vi "GDI Resize Image.vi"(7 "Image Data":T1, 8 "error in (no error)":errorcluster, 9 "Height":i32=400, 10 "Width":i32=800, 11 "Path":path) -> (0 "error out":errorcluster, 3 "Resized image data":T1)   [LabVIEW 2011]
doc: "Use the Windows GDI functions to resize an image."
uses:
  <vilib>/picture/picture.llb/imagedata.ctl
  System.Drawing
  <vilib>/Utility/colorconv.llb/Color to RGB.vi
  <vilib>/wsapi/NI_WebServices.lvlib
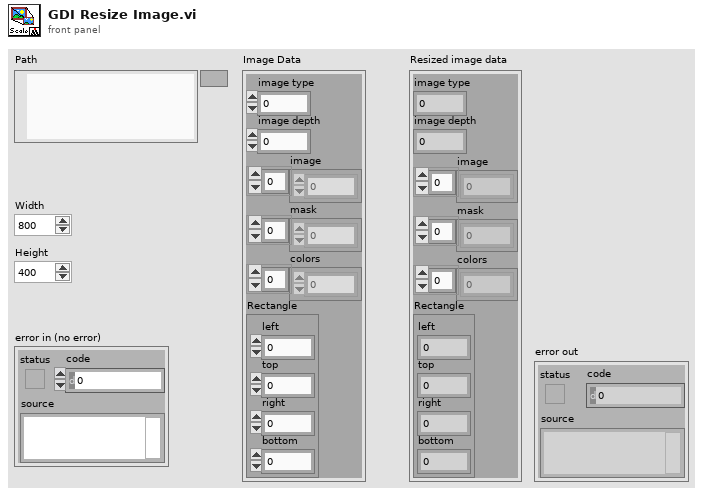
[diagram p1: front panel]
types:
  T1 = typedef "imagedata.ctl" = cluster{"image type":i32, "image depth":i32, "image":u8[], "mask":u8[], "colors":u32[], "Rectangle":cluster{"left":i16, "top":i16, "right":i16, "bottom":i16}}
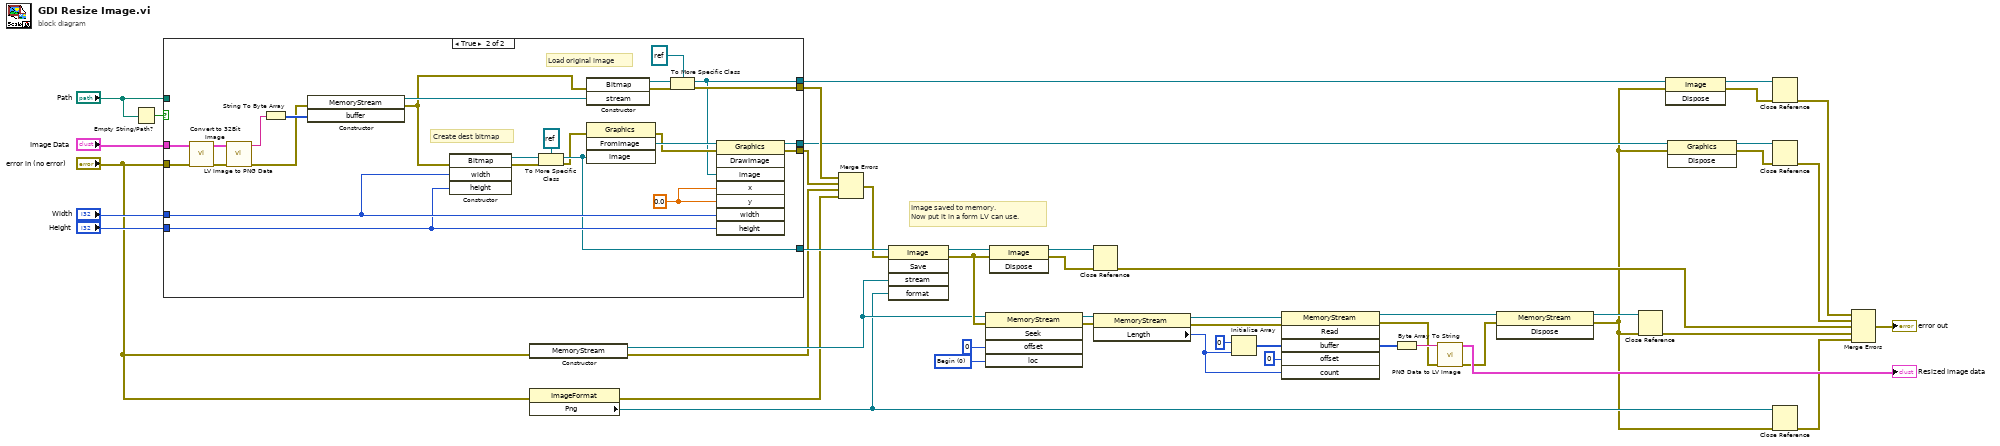
[diagram p0: block diagram]
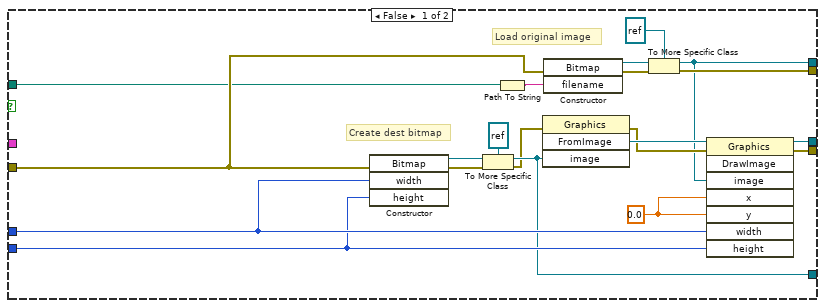
[diagram p2: hidden frame]
diagram:
  w42 = 0 items=["Begin", "Current", "End"] ("loc")
  # "Image saved to memory. \nNow put it in a form LV can use."
  n1 = Empty String/Path?(string/path="Path") -> (empty?=w2:bool)
  n2 = case shown="True" w2 {
    tunnel: "Width" -> [w64 w90]
    tunnel: "Height" -> [w63 w89]
    tunnel: [w62 w88] -> w32
    tunnel: [w58 w84] -> w30
    tunnel: [w53 w80] -> w28
    tunnel: [w52 w79] -> w27
    tunnel: [w51 w78] -> w22
    tunnel: "error in (no error)" -> [w50 w73]
    tunnel: "Path" -> [w49 _]
    tunnel: "Image Data" -> [_ w72]
    frame False {
      w68 = sgl 0.0 ("x")
      # "Create dest bitmap"
      # "Load original image"
      n3 = constructor class="Bitmap"(error in=w50, "width"=w64, "height"=w63) -> (reference out=w66:refnum<k24>, error out=w61:errorcluster)  [unwired: 2 in, 3 out]
      n4 = To More Specific Class(target class=refnum<k24> refnum, reference=w66, error in=w61) -> (specific class reference=w62:refnum<k24>, error out=w60:errorcluster)
      n5 = Path To String(path=w49) -> (string=w57:string)
      n6 = invoke class="Graphics" method="FromImage"(error in=w60, "image"=w62) -> (error out=w59:errorcluster, "FromImage"=w65:refnum<k24>)  [unwired: 2 in, 2 out]
      n7 = constructor class="Bitmap"(error in=w50, "filename"=w57) -> (reference out=w55:refnum<k24>, error out=w54:errorcluster)  [unwired: 2 in, 2 out]
      n8 = To More Specific Class(target class=refnum<k24> refnum, reference=w55, error in=w54) -> (specific class reference=w52:refnum<k24>, error out=w53:errorcluster)
      n9 = invoke class="Graphics" method="DrawImage"(reference=w65, error in=w59, "image"=w52, "x"=w68, "y"=w68, "width"=w64, "height"=w63) -> (reference out=w51:refnum<k24>, error out=w58:errorcluster)  [unwired: 1 in, 6 out]
    }
    frame True {
      w94 = sgl 0.0 ("x")
      # "Create dest bitmap"
      # "Load original image"
      n10 = call "Convert to 32Bit Image.vi"("error in (no error)"=w73, "Image Data"=w72) -> ("error out"=w77:errorcluster, "32Bit Image Data Out"=w76:T1)  [unwired: 8 in]
      n11 = call <vilib>:"LV Image to PNG Data.vi"("error in (no error)"=w77, "image data"=w76) -> ("error out"=w69:errorcluster, "png data"=w75:string)  [unwired: 8 in]
      n12 = String To Byte Array(string=w75) -> (unsigned byte array=w74:u8[])
      n13 = constructor class="MemoryStream"(error in=w69, "buffer"=w74) -> (reference out=w71:refnum<k24>, error out=w70:errorcluster)  [unwired: 2 in, 2 out]
      n14 = constructor class="Bitmap"(error in=w70, "width"=w90, "height"=w89) -> (reference out=w92:refnum<k24>, error out=w87:errorcluster)  [unwired: 2 in, 3 out]
      n15 = To More Specific Class(target class=refnum<k24> refnum, reference=w92, error in=w87) -> (specific class reference=w88:refnum<k24>, error out=w86:errorcluster)
      n16 = invoke class="Graphics" method="FromImage"(error in=w86, "image"=w88) -> (error out=w85:errorcluster, "FromImage"=w91:refnum<k24>)  [unwired: 2 in, 2 out]
      n17 = constructor class="Bitmap"(error in=w70, "stream"=w71) -> (reference out=w82:refnum<k24>, error out=w81:errorcluster)  [unwired: 2 in, 2 out]
      n18 = To More Specific Class(target class=refnum<k24> refnum, reference=w82, error in=w81) -> (specific class reference=w79:refnum<k24>, error out=w80:errorcluster)
      n19 = invoke class="Graphics" method="DrawImage"(reference=w91, error in=w85, "image"=w79, "x"=w94, "y"=w94, "width"=w90, "height"=w89) -> (reference out=w78:refnum<k24>, error out=w84:errorcluster)  [unwired: 1 in, 6 out]
    }
  }
  n20 = constructor class="MemoryStream"(error in="error in (no error)") -> (reference out=w29:refnum<k24>, error out=w12:errorcluster)  [unwired: 2 in, 1 out]
  n21 = property class="ImageFormat"(error in="error in (no error)") -> (error out=w11:errorcluster, "Png"=w20:refnum<k24>)  [unwired: 1 in, 1 out]
  n22 = Merge Errors(w28, w30, w12, w11) -> (w23:errorcluster)
  n23 = invoke class="Image" method="Save"(reference=w32, error in=w23, "stream"=w29, "format"=w20) -> (reference out=w46:refnum<k24>, error out=w34:errorcluster)  [unwired: 1 in, 3 out]
  n24 = invoke class="MemoryStream" method="Seek"(reference=w29, error in=w34, "offset"=i64 0, "loc"=w42) -> (reference out=w45:refnum<k24>, error out=w44:errorcluster)  [unwired: 1 in, 3 out]
  n25 = invoke class="Image" method="Dispose"(reference=w46, error in=w34) -> (reference out=w24:refnum<k24>, error out=w18:errorcluster)  [unwired: 1 in, 1 out]
  n26 = Close Reference(reference=w24, error in (no error)=w18) -> (error out=w15:errorcluster)
  n27 = property class="MemoryStream"(reference=w45, error in=w44) -> (reference out=w40:refnum<k24>, error out=w39:errorcluster, "Length"=w37:i64)
  n28 = Initialize Array(u8 0 ("element"), w37) -> (w38:u8[])
  n29 = invoke class="MemoryStream" method="Read"(reference=w40, error in=w39, "buffer"=w38, "offset"=0, "count"=w37) -> (reference out=w35:refnum<k24>, error out=w17:errorcluster, "buffer"=w33:u8[])  [unwired: 1 in, 3 out]
  n30 = Byte Array To String(unsigned byte array=w33) -> (string=w31:string)
  n31 = call <vilib>:"PNG Data to LV Image.vi"("error in (no error)"=w17, "png data"=w31) -> ("error out"=w16:errorcluster, "image data"=→"Resized image data":T1)  [unwired: 8 in]
  n32 = invoke class="MemoryStream" method="Dispose"(reference=w35, error in=w16) -> (reference out=w26:refnum<k24>, error out=w10:errorcluster)  [unwired: 1 in, 1 out]
  n33 = Close Reference(reference=w26, error in (no error)=w10) -> (error out=w14:errorcluster)
  n34 = invoke on="Release the file lock" class="Image" method="Dispose"(reference=w27, error in=w10) -> (reference out=w25:refnum<k24>, error out=w8:errorcluster)  [unwired: 1 in, 1 out]
  n35 = invoke class="Graphics" method="Dispose"(reference=w22, error in=w10) -> (reference out=w21:refnum<k24>, error out=w9:errorcluster)  [unwired: 1 in, 1 out]
  n36 = Close Reference(reference=w25, error in (no error)=w8) -> (error out=w5:errorcluster)
  n37 = Close Reference(reference=w21, error in (no error)=w9) -> (error out=w6:errorcluster)
  n38 = Close Reference(reference=w20, error in (no error)=w10) -> (error out=w7:errorcluster)
  n39 = Merge Errors(w5, w6, w15, w14, w7) -> (→"error out":errorcluster)
